vi "Set_Daxsonics_BP2.vi"(5 "VISA resource name":refnum<visa-resource-name>="COM8", 8 "Number of Channels":i32=5, 9 "Daxsonics Settings":T1={"Freq (MHz) "=20, "Voltage (V)"=0, "Gain (dB)"=22} {"Freq (MHz)" items=["4"=4, "6"=6, "8"=8, "10"=10, "12"=12, "15"=15, "17"=17, "20"=20, "25"=25, "30"=30, "35"=35, "40"=40, "45"=45, "50"=50]; "Voltage (V)" items=["0"=0, "10"=10, "20"=20, "30"=30, "40"=40, "50"=50, "60"=60, "70"=70, "80"=80, "90"=90, "100"=100, "110"=110, "120"=120, "130"=130, "140"=140, "150"=150, "160"=160, "170"=170, "180"=180, "190"=190]; "Gain (dB)" items=["22"=22, "25"=25, "28"=28, "31"=31, "34"=34, "37"=37, "40"=40, "43"=43, "46"=46, "49"=49, "52"=52, "55"=55, "58"=58, "61"=61, "64"=64]}) -> ()   [LabVIEW 2022 SP3]
doc: "This application VI allows the user to set the desired parameters in the \n5800 / 5900 P / R. just select thevalues that you want to set the instrument to from the 5800 / 5900 user interface and click on the send to 5800 button."
uses:
  ScanningControl/Motion Controllers/-MotionRoutines/MotionGlobals.vi
  ScanningControl/Pulsers/Daxsonics/-DaxSubroutines/Dax_Control_Cluster.ctl
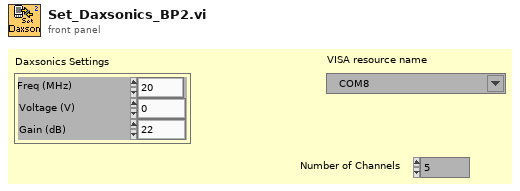
[diagram p1: front panel]
types:
  T1 = typedef "Dax_Control_Cluster.ctl" = cluster{"Freq (MHz) ":u16, "Voltage (V)":u16, "Gain (dB)":u16}
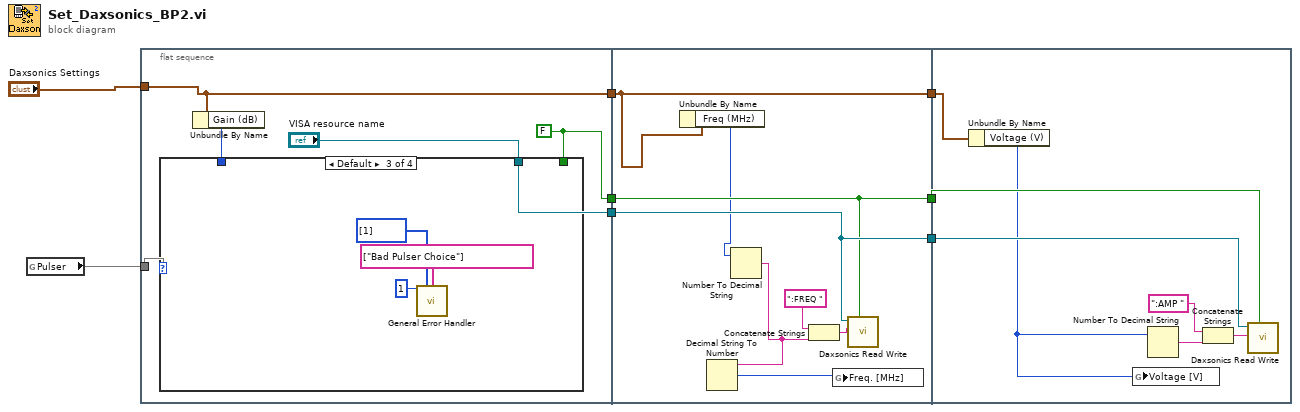
[diagram p0: block diagram]
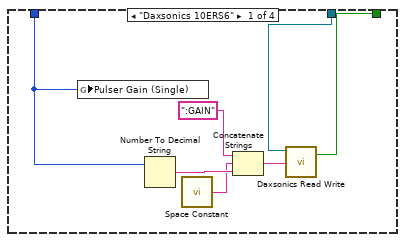
[diagram p2: hidden frame]
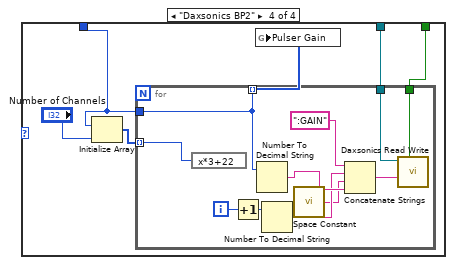
[diagram p4: hidden frame]
diagram:
  n1 = global read "MotionGlobals.vi" "Pulser"() -> (w1)
  n2 = flat-sequence {
    tunnel: ["VISA resource name"] -> w7
    tunnel: [w10] -> w6
    tunnel: "Daxsonics Settings" -> [w12]
    tunnel: [w12] -> w4
    tunnel: w1 -> [w9]
    tunnel: [w45] -> w8
    tunnel: w7 -> [w45]
    tunnel: w6 -> [w44]
    tunnel: [w44] -> w5
    tunnel: w4 -> [w42]
    tunnel: [w42] -> w3
    tunnel: w8 -> [w52]
    tunnel: w5 -> [w51]
    tunnel: w3 -> [w50]
    frame #0 {
      w10 = FALSE ("Enable Termination\nChar (T)")
      n3 = Unbundle By Name(w12) -> ("Gain (dB)"=w11:u16)
      n4 = case shown="Default" w9 {
        tunnel: "VISA resource name" -> [w15 _ _ w26]
        tunnel: w11 -> [w16 _ _ w25]
        tunnel: w10 -> [w14 _ _ w24]
        frame "Daxsonics 10ERS6" {
          n5 = global write "MotionGlobals.vi" "Pulser Gain (Single)"(w16) -> ()
          n6 = Number To Decimal String(number=w16) -> (decimal integer string=w20:string)  [unwired: 1 in]
          n7 = call <vilib>:"Space Constant.vi"() -> ("String"=w17:string)
          n8 = Concatenate Strings(":GAIN" ("string"), w17, w20) -> (w19:string)
          n9 = call "Daxsonics Read Write.vi"("Daxsonics Name"=w14, "write buffer"=w19, "VISA resource name"=w15) -> ()  [unwired: 6 in, 3 out]
        }
        frame "Daxsonics BP1" {
        }
        frame Default {
          n10 = call <vilib>:"General Error Handler.vi"("[error code] (0)"=1, "[user-defined codes]"=i32[] [1], "[user-defined descriptions]"=string[] ["Bad Pulser Choice"]) -> ()  [unwired: 8 in, 5 out]
        }
        frame "Daxsonics BP2" {
          n11 = Initialize Array(w25, "Number of Channels") -> (w28:u16[])
          n12 = for {
            tunnel: w26 -> [w37]
            tunnel: w24 -> [w33]
            tunnel: w28 -> [w31] mode=indexing
            tunnel: [w30] -> w27 mode=indexing
            tunnel: w25 -> [w30]
            i -> [w36]
            n13 = expression code="x*3+22"(w31) -> ()  [unwired: 1 out]
            n14 = Increment(x=w36) -> (x+1=w32:i32)
            n15 = Number To Decimal String(number=w30) -> (decimal integer string=w40:string)  [unwired: 1 in]
            n16 = Number To Decimal String(number=w32) -> (decimal integer string=w35:string)  [unwired: 1 in]
            n17 = call <vilib>:"Space Constant.vi"() -> ("String"=w34:string)
            n18 = Concatenate Strings(":GAIN" ("string"), w35, w34, w40) -> (w39:string)
            n19 = call "Daxsonics Read Write.vi"("Daxsonics Name"=w33, "write buffer"=w39, "VISA resource name"=w37) -> ()  [unwired: 6 in, 3 out]
          }
          n20 = global write "MotionGlobals.vi" "Pulser Gain"(w27) -> ()
        }
      }
    }
    frame #1 {
      n21 = Unbundle By Name(w42) -> ("Freq (MHz)"=w41:u16)
      n22 = Number To Decimal String(number=w41) -> (decimal integer string=w43:string)  [unwired: 1 in]
      n23 = Decimal String To Number(string=w43) -> (number=w46:i32)  [unwired: 2 in, 1 out]
      n24 = Concatenate Strings(":FREQ " ("string"), w43) -> (w48:string)
      n25 = global write "MotionGlobals.vi" "Freq. [MHz]"(w46) -> ()
      n26 = call "Daxsonics Read Write.vi"("Daxsonics Name"=w44, "write buffer"=w48, "VISA resource name"=w45) -> ()  [unwired: 6 in, 3 out]
    }
    frame #2 {
      n27 = Unbundle By Name(w50) -> ("Voltage (V)"=w49:u16)
      n28 = global write "MotionGlobals.vi" "Voltage [V]"(w49) -> ()
      n29 = Number To Decimal String(number=w49) -> (decimal integer string=w55:string)  [unwired: 1 in]
      n30 = Concatenate Strings(":AMP " ("string"), w55) -> (w54:string)
      n31 = call "Daxsonics Read Write.vi"("Daxsonics Name"=w51, "write buffer"=w54, "VISA resource name"=w52) -> ()  [unwired: 6 in, 3 out]
    }
  }
